vi "PLC_OP30_Read.vi"(8 "error in (no error)":errorcluster, 11 "S7 Connection in":T1) -> (0 "error out":errorcluster, 3 "S7 Connection out 2":T1)   [LabVIEW 2017]
uses:
  <vilib>/DATA AHEAD/SP7/typedefs/S7 Connection.ctl
  <vilib>/DATA AHEAD/SP7/typedefs/PLC Type.ctl
  <vilib>/DATA AHEAD/SP7/functions/read/read Dint array.vi
  <vilib>/DATA AHEAD/SP7/functions/read/read real array.vi
  <vilib>/DATA AHEAD/SP7/functions/read/read String.vi
  <vilib>/DATA AHEAD/SP7/SP7.lvlib
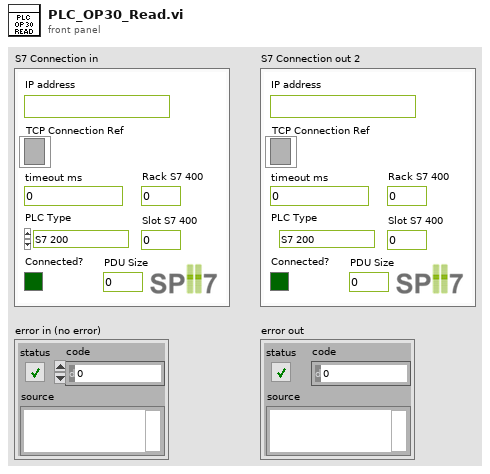
[diagram p1: front panel]
types:
  T1 = typedef "SP7.lvlib/S7 Connection.ctl" = cluster{"TCP Connection Ref":refnum<k5>, "IP address":string, "timeout ms":i32, "Connected?":bool, "PLC Type":T2, "Rack S7 400":u8, "Slot S7 400":u8, "PDU Size":u16, "connection semaphore":T3}
  T2 = typedef "SP7.lvlib/PLC Type.ctl" = enum16{"S7 200", "S7 300/400", "S7 1200", "S7 1500", "LOGO!8"}
  T3 = typedef "Semaphore RefNum" = refnum<k1>
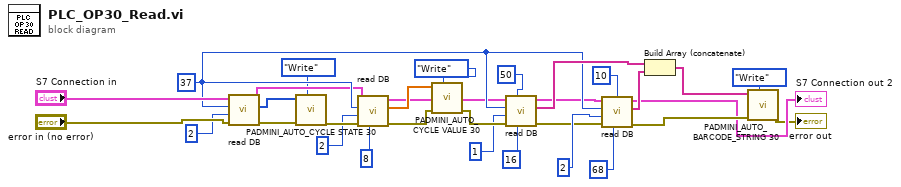
[diagram p0: block diagram]
diagram:
  w26 = u16 37 ("Data Block #")
  n1 = call-poly <vilib>:"read DB.vi"("error in (no error)"="error in (no error)", "items #"=u16 2 ("Items # [byte]"), "Data Block #"=w26, "S7 Connection in"="S7 Connection in") -> ("error out"=w2:errorcluster, "DINT result array"=w4:i32[], "S7 Connection out"=w7:T1)  [unwired: 5 in]
  n2 = call "PADMINI_AUTO_CYCLE STATE 30.vi"("Enum"=enum16{"Read", "Write"}."Write", "error in (no error)"=w2, "Input"=w4) -> ("error out"=w6:errorcluster)  [unwired: 7 in, 1 out]
  n3 = call-poly <vilib>:"read DB.vi"("Item offset [byte]"=u32 8, "error in (no error)"=w6, "items #"=u16 2 ("Items # [byte]"), "Data Block #"=w26, "S7 Connection in"=w7) -> ("error out"=w14:errorcluster, "REAL result array"=w16:sgl[], "S7 Connection out"=w8:T1)  [unwired: 4 in]
  n4 = call "PADMINI_AUTO_CYCLE VALUE 30.vi"("Enum"=enum16{"Read", "Write"}."Write", "error in (no error)"=w14, "Input"=w16) -> ("error out"=w15:errorcluster)  [unwired: 7 in, 1 out]
  n5 = call-poly <vilib>:"read DB.vi"("Item offset [byte]"=u32 16, "String length reserved in DB (default=254)"=u32 50 ("Item offset [byte]"), "error in (no error)"=w15, "items #"=u16 1 ("Items # [byte]"), "Data Block #"=w26, "S7 Connection in"=w8) -> ("error out"=w20:errorcluster, "STRING result Array"=w27:string[], "S7 Connection out"=w21:T1)  [unwired: 2 in, 1 out]
  n6 = call-poly <vilib>:"read DB.vi"("Item offset [byte]"=u32 68, "String length reserved in DB (default=254)"=u32 10 ("Item offset [byte]"), "error in (no error)"=w20, "items #"=u16 2 ("Items # [byte]"), "Data Block #"=w26, "S7 Connection in"=w21) -> ("error out"=w19:errorcluster, "STRING result Array"=w29:string[], "S7 Connection out"=→"S7 Connection out 2":T1)  [unwired: 2 in, 1 out]
  n7 = Build Array (concatenate)(w27, w29) -> (w28:string[])
  n8 = call "PADMINI_AUTO_BARCODE_STRING 30.vi"("Enum"=enum16{"Read", "Write"}."Write", "error in (no error)"=w19, "Input"=w28) -> ("error out"=→"error out":errorcluster)  [unwired: 7 in, 1 out]
